vi "ConnectedAxes.vi"() -> ()   [LabVIEW 2010]
panel:
  out "Conn. Axes":string[](array[string])
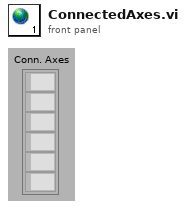
[diagram p1: front panel]
diagram:
